vi "Draw.vi"(8 "Error In":errorcluster, 9 "Coordinants":cluster{"X":i16, "Y":i16}, 10 "2D Picture In":picture, 11 "Rectangle in":refnum<class "Rectangle.lvclass">) -> (0 "Error Out":errorcluster, 2 "2D Picture Out":picture, 3 "Rectangle out":refnum<class "Rectangle.lvclass">)   [LabVIEW 2021, in "Rectangle.lvclass"]
doc: "Draw a rectangle on 2D picture.\nCoordinates is positison of left upper corner of this figure."
uses:
  Rectangle.lvclass
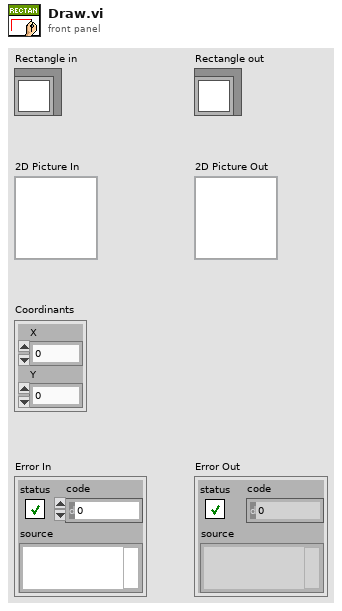
[diagram p1: front panel]
types:
  T1 = cluster{"left":i16, "top":i16, "right":i16, "bottom":i16}
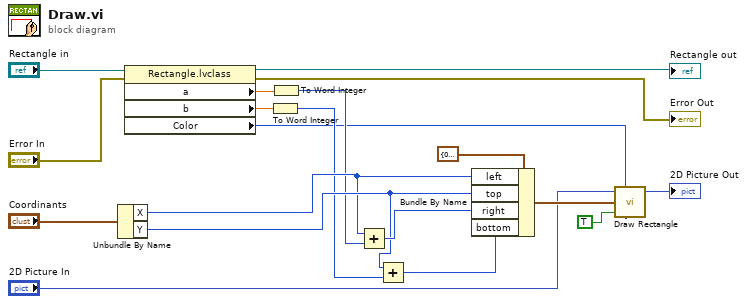
[diagram p0: block diagram]
diagram:
  n1 = Unbundle By Name("Coordinants") -> ("X"=w10:i16, "Y"=w11:i16)
  n2 = property class="Rectangle.lvclass"(reference="Rectangle in", error in="Error In") -> (reference out=→"Rectangle out":refnum<class "Rectangle.lvclass">, error out=→"Error Out":errorcluster, "a"=w13:dbl, "b"=w12:dbl, "Color"=w2:u32)
  n3 = To Word Integer(number=w12) -> (16bit integer=w8:i16)
  n4 = To Word Integer(number=w13) -> (16bit integer=w9:i16)
  n5 = Add(x=w10, y=w9) -> (x+y=w17:i16)
  n6 = Add(x=w11, y=w8) -> (x+y=w16:i16)
  n7 = Bundle By Name(cluster=T1 {"left"=0, "top"=0, "right"=0, "bottom"=0} ("rect"), "left"=w10, "top"=w11, "right"=w17, "bottom"=w16) -> (w4:T1)
  n8 = call <vilib>:"Draw Rectangle.vi"("picture"="2D Picture In", "rect"=w4, "fill?(F)"=TRUE, "color(black)"=w2) -> ("new picture"=→"2D Picture Out":picture)  [unwired: 5 in]
